vi "Message Handling Loop - Data.vi"(8 "error in":errorcluster, 9 "Queue in":refnum<queue>, 10 "User Event - Stop":refnum<user-event>) -> (0 "error out":errorcluster)   [LabVIEW 2018]
uses:
  Support/Message Queue/Message Cluster.ctl
  Type Defs/Data Loop Data.ctl
  Support/Message Queue/Enqueue Message (Single).vi
  <vilib>/Utility/error.llb/Error Cluster From Error Code.vi
  <vilib>/ErrorRing/Error Ring.xnode
  Support/Message Queue/Message Queue.lvlib
  Support/User Event - Stop/User Event - Stop.lvlib
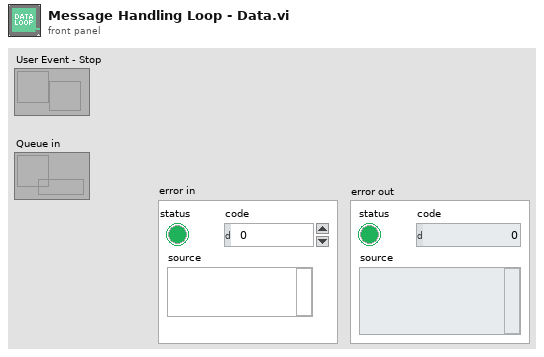
[diagram p1: front panel]
types:
  T1 = typedef "Data Loop Data.ctl" = cluster{"Update List":i32[], "File Path":path, "Refresh SRs":refnum<vi>, "Add SR":refnum<vi>}
  T2 = typedef "SR Cluster.ctl" = cluster{"Color":u32, "SR Number":i32, "SR Status":T3, "SR Type":string, "Summary":string, "Last Updated":timestamp, "Service Level":string, "Days Open":dbl, "Creation Date":timestamp}
  T3 = typedef "SR Status.ctl" = enum16{"Caller Abandoned", "Created in Error", "Expired", "Forum Resolved AE", "Forum Resolved Customer", "IN WORK", "IN WORK Collab with AES", "IN WORK Collab with PSE", "IN WORK Collab with SE", "IN WORK Customer Added Note", "IN WORK Escalation", "IN WORK Wait on Customer", "Open", "Potentially Resolved", "Presumed Resolved", "RMA Approved for Return", "Resolved", "Passed Off"}
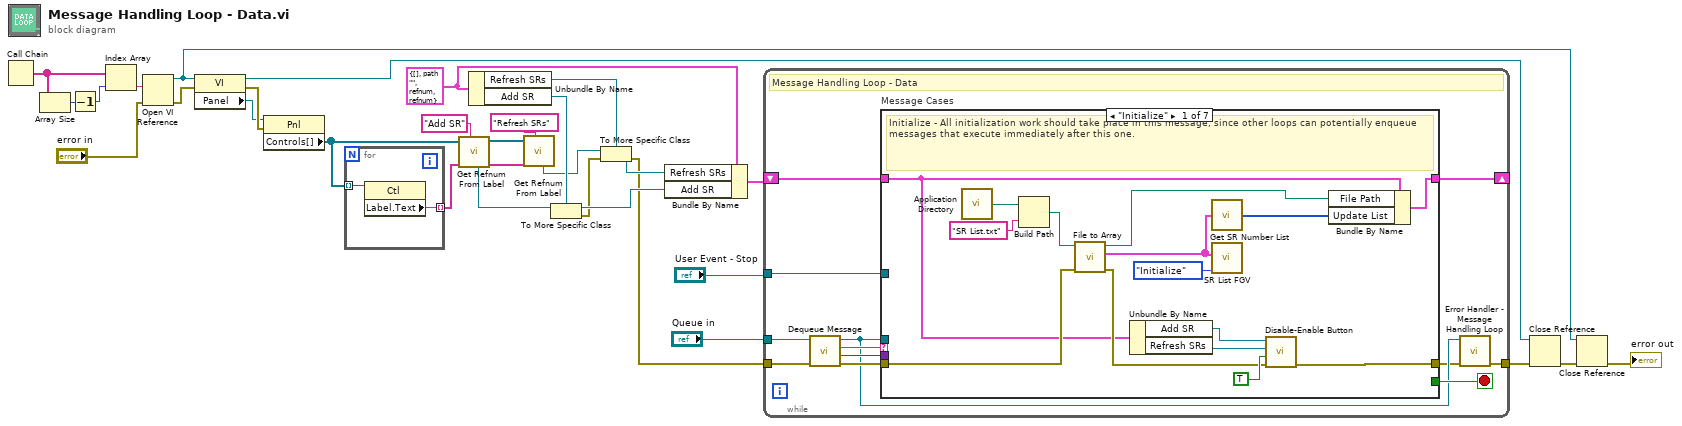
[diagram p0: block diagram]
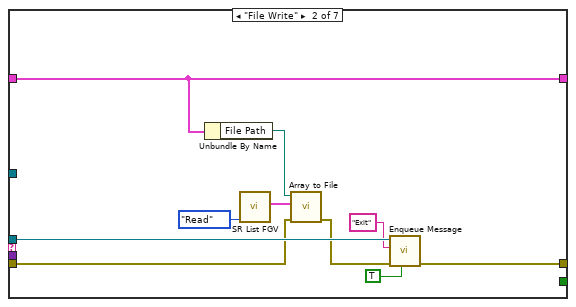
[diagram p2: hidden frame]
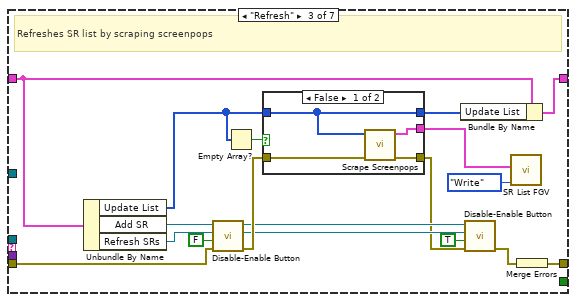
[diagram p3: hidden frame]
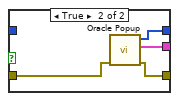
[diagram p4: hidden frame]
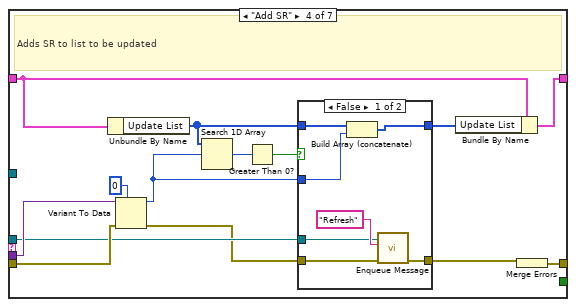
[diagram p5: hidden frame]
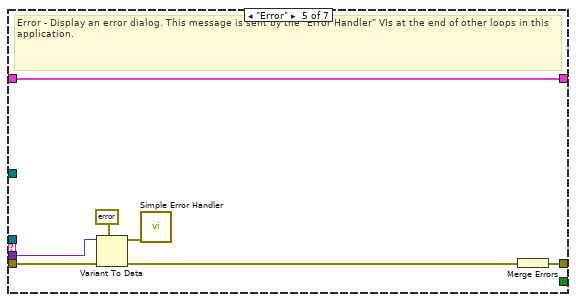
[diagram p7: hidden frame]
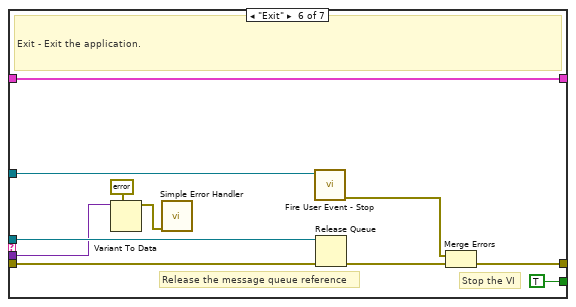
[diagram p8: hidden frame]
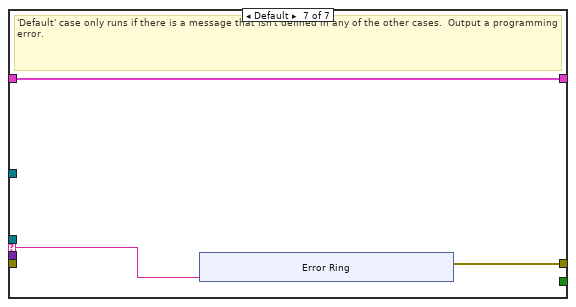
[diagram p9: hidden frame]
diagram:
  w9 = T1 {"Update List"=[], "File Path"=path "", "Refresh SRs"=refnum, "Add SR"=refnum} ("Data Loop Data")
  n1 = Call Chain() -> (call chain=w29:string[])
  n2 = Array Size(array=w29) -> (size(s)=w28:i32)
  n3 = Decrement(x=w28) -> (x-1=w27:i32)
  n4 = Index Array(array=w29, index=w27) -> (element=w26:string)
  n5 = Open VI Reference(vi path=w26, error in (no error)="error in") -> (vi reference=w5:refnum<vi>, error out=w14:errorcluster)  [unwired: 4 in]
  n6 = property class="VI"(reference=w5, error in=w14) -> (reference out=w7:refnum<vi>, error out=w13:errorcluster, "Panel"=w12:refnum<vi>)
  n7 = property class="Pnl"(reference=w12, error in=w13) -> ("Controls[]"=w25:refnum<vi>[])  [unwired: 2 out]
  n8 = for {
    tunnel: w25 -> [w33] mode=indexing
    tunnel: [w32] -> w24 mode=indexing
    n9 = property class="Ctl"(reference=w33) -> ("Label.Text"=w32:string)  [unwired: 1 in, 2 out]
  }
  n10 = call "Get Refnum From Label.vi"("label"="Add SR", "label array in"=w24, "controls[] in"=w25) -> ("label array out"=w22:string[], "controls[] out"=w23:refnum<vi>[], "refnum out"=w17:refnum<vi>)  [unwired: 6 in]
  n11 = Unbundle By Name(w9) -> ("Refresh SRs"=w21:refnum<vi>, "Add SR"=w18:refnum<vi>)
  n12 = call "Get Refnum From Label.vi"("label"="Refresh SRs", "label array in"=w22, "controls[] in"=w23) -> ("refnum out"=w15:refnum<vi>)  [unwired: 6 in, 2 out]
  n13 = To More Specific Class(target class=w18, reference=w17) -> (specific class reference=w19:refnum<vi>, error out=w16:errorcluster)  [unwired: 1 in]
  n14 = To More Specific Class(target class=w21, reference=w15, error in=w16) -> (specific class reference=w20:refnum<vi>, error out=w1:errorcluster)
  n15 = Bundle By Name(cluster=w9, "Refresh SRs"=w20, "Add SR"=w19) -> (w8:T1)
  n16 = while {
    tunnel: "Queue in" -> [w41]
    tunnel: [w39] -> w6
    tunnel: "User Event - Stop" -> [w37]
    shift-right: [w35] -> _
    shift-left: w8 -> [w36]
    tunnel: w1 -> [w34]
    stop <- w45 stop-if-true
    # "Message Handling Loop - Data"
    n17 = call "Dequeue Message.vi"("error in (no error)"=w34, "Message Queue"=w41) -> ("error out"=w44:errorcluster, "Message Data"=w42:variant, "Message"=w43:string, "dup Message Queue"=w40:refnum<queue>)  [unwired: 6 in]
    n18 = case "Message Cases" shown="\"Initialize\"" w43 {
      selector: w43 -> [_ _ _ _ _ _ w139]
      tunnel: w40 -> [_ w70 _ w99 _ w137 _]
      tunnel: w44 -> [w55 w65 w85 w106 w126 w132 _]
      tunnel: [w51 w69 w88 w110 w121 w134 w140] -> w38
      tunnel: [_ _ _ _ _ TRUE _] -> w45
      tunnel: w42 -> [_ _ _ w107 w125 w129 _]
      tunnel: w37 -> [_ _ _ _ _ w128 _]
      tunnel: w36 -> [w48 w62 w73 w109 w120 w127 w138]
      tunnel: [w59 w62 w72 w108 w120 w127 w138] -> w35
      frame "Initialize" {
        # "Initialize - All initialization work should take place in this message, since other loops can potentially enqueue messages that execute immediately after this one."
        n19 = call <vilib>:"Application Directory.vi"() -> ("Application Directory"=w58:path)
        n20 = Build Path(base path=w58, name or relative path="SR List.txt") -> (appended path=w54:path)
        n21 = call "File to Array.vi"("error in"=w55, "file path in"=w54) -> ("error out"=w49:errorcluster, "list out"=w52:T2[], "file path out"=w53:path)  [unwired: 7 in]
        n22 = Unbundle By Name(w48) -> ("Add SR"=w47:refnum<vi>, "Refresh SRs"=w46:refnum<vi>)
        n23 = call "Get SR Number List.vi"("list in"=w52) -> ("SR number array out"=w56:i32[])  [unwired: 4 in]
        n24 = call "SR List FGV.vi"("Operation"=enum16{"Initialize", "Write", "Read", "Clear"}."Initialize", "list in"=w52) -> ()  [unwired: 8 in, 2 out]
        n25 = call "Disable-Enable Button.vi"("error in"=w49, "Enabled?"=TRUE, "Refresh SRs in"=w46, "Add SR in"=w47) -> ("error out"=w51:errorcluster)  [unwired: 5 in, 2 out]
        n26 = Bundle By Name(cluster=w48, "File Path"=w53, "Update List"=w56) -> (w59:T1)
      }
      frame "File Write" {
        n27 = Unbundle By Name(w62) -> ("File Path"=w61:path)
        n28 = call "SR List FGV.vi"("Operation"=enum16{"Initialize", "Write", "Read", "Clear"}."Read") -> ("list out"=w64:T2[])  [unwired: 9 in, 1 out]
        n29 = call "Array to File.vi"("error in"=w65, "array in"=w64, "file path in"=w61) -> ("error out"=w66:errorcluster)  [unwired: 7 in, 1 out]
        n30 = call-poly "Enqueue Message.vi"("Priority Message? (F)"=TRUE, "error in (no error)"=w66, "Message"="Exit", "Message Queue"=w70) -> ("error out"=w69:errorcluster)  [unwired: 6 in, 1 out]
      }
      frame "Refresh" {
        # "Refreshes SR list by scraping screenpops"
        n31 = Unbundle By Name(w73) -> ("Update List"=w74:i32[], "Add SR"=w87:refnum<vi>, "Refresh SRs"=w86:refnum<vi>)
        n32 = call "Disable-Enable Button.vi"("error in"=w85, "Enabled?"=FALSE, "Refresh SRs in"=w86, "Add SR in"=w87) -> ("error out"=w84:errorcluster, "Refresh SRs out"=w81:refnum<vi>, "Add SR out"=w82:refnum<vi>)  [unwired: 5 in]
        n33 = Empty Array?(array=w74) -> (empty?=w75:bool)
        n34 = case shown="False" w75 {
          tunnel: w74 -> [w89 _]
          tunnel: w84 -> [w91 w95]
          tunnel: [w92 w94] -> w77
          tunnel: [w90 w96] -> w76
          tunnel: [w89 w93] -> w71
          frame False {
            n35 = call "Scrape Screenpops.vi"("error in"=w91, "SR number list in"=w89) -> ("error out"=w90:errorcluster, "sr clusters out"=w92:T2[])  [unwired: 8 in]
          }
          frame True {
            n36 = call "Oracle Popup.vi"("error in"=w95) -> ("error out"=w96:errorcluster, "SR List out"=w94:T2[], "SR number list out"=w93:i32[])  [unwired: 8 in]
          }
        }
        n37 = Bundle By Name(cluster=w73, "Update List"=w71) -> (w72:T1)
        n38 = call "Disable-Enable Button.vi"("error in"=w76, "Enabled?"=TRUE, "Refresh SRs in"=w81, "Add SR in"=w82) -> ("error out"=w80:errorcluster)  [unwired: 5 in, 2 out]
        n39 = call "SR List FGV.vi"("Operation"=enum16{"Initialize", "Write", "Read", "Clear"}."Write", "list in"=w77) -> ()  [unwired: 8 in, 2 out]
        n40 = Merge Errors(w80) -> (w88:errorcluster)
      }
      frame "Add SR" {
        # "Adds SR to list to be updated"
        n41 = Unbundle By Name(w109) -> ("Update List"=w101:i32[])
        n42 = Variant To Data(error in=w106, type=0, Variant=w107) -> (data=w100:i32, error out=w97:errorcluster)
        n43 = Search 1D Array(1D array=w101, element=w100) -> (index of element=w104:i32)  [unwired: 1 in]
        n44 = Greater Than 0?(x=w104) -> (x > 0?=w103:bool)
        n45 = case shown="False" w103 {
          tunnel: [w116 w119] -> w102
          tunnel: w101 -> [w117 w119]
          tunnel: w100 -> [w115 _]
          tunnel: w99 -> [w113 _]
          tunnel: [w112 w118] -> w98
          tunnel: w97 -> [w111 w118]
          frame False {
            n46 = Build Array (concatenate)(w117, w115) -> (w116:i32[])
            n47 = call-poly "Enqueue Message.vi"("error in (no error)"=w111, "Message"="Refresh", "Message Queue"=w113) -> ("error out"=w112:errorcluster)  [unwired: 7 in, 1 out]
          }
          frame True {
          }
        }
        n48 = Bundle By Name(cluster=w109, "Update List"=w102) -> (w108:T1)
        n49 = Merge Errors(w98) -> (w110:errorcluster)
      }
      frame "Error" {
        # "Error - Display an error dialog. This message is sent by the \"Error Handler\" VIs at the end of other loops in this application."
        n50 = Variant To Data(error in=w126, type=errorcluster {"status"=FALSE, "code"=0, "source"=""} ("error constant"), Variant=w125) -> (data=w123:errorcluster, error out=w122:errorcluster)
        n51 = call <vilib>:"Simple Error Handler.vi"("error in (no error)"=w123) -> ()  [unwired: 4 in, 5 out]
        n52 = Merge Errors(w122) -> (w121:errorcluster)
      }
      frame "Exit" {
        # "Stop the VI"
        # "Release the message queue reference"
        # "Exit - Exit the application."
        n53 = Variant To Data(type=errorcluster {"status"=FALSE, "code"=0, "source"=""} ("error constant"), Variant=w129) -> (data=w130:errorcluster)  [unwired: 1 in, 1 out]
        n54 = call <vilib>:"Simple Error Handler.vi"("error in (no error)"=w130) -> ()  [unwired: 4 in, 5 out]
        n55 = call "Fire User Event - Stop.vi"("User Event - Stop"=w128) -> ("error out"=w133:errorcluster)  [unwired: 10 in]
        n56 = Release Queue(queue=w137, error in (no error)=w132) -> (error out=w135:errorcluster)  [unwired: 1 in, 2 out]
        n57 = Merge Errors(w133, w135) -> (w134:errorcluster)
      }
      frame Default {
        # "'Default' case only runs if there is a message that isn't defined in any of the other cases.  Output a programming error."
        n58 = xnode "Error Ring"("parameter 0"=w139) -> ("error out"=w140:errorcluster)
      }
    }
    n59 = call "Error Handler - Message Handling Loop.vi"("error in (no error)"=w38, "Message Queue"=w40) -> ("dup error in"=w39:errorcluster)  [unwired: 8 in, 1 out]
  }
  n60 = Close Reference(reference=w7, error in (no error)=w6) -> (error out=w4:errorcluster)
  n61 = Close Reference(reference=w5, error in (no error)=w4) -> (error out=→"error out":errorcluster)
